vi "36DUT Plot Subvi Ver1.0.vi"(6 "Plot":T1(ring), 7 "No of Rows":i32=10496, 8 "error in (no error)":errorcluster, 9 "No of DUT":i32=16, 10 "Bank":enum16{"C1", "C2", "C3"}(ring), 11 "file path (dialog if empty)":path) -> (0 "error out":errorcluster, 3 "Delta C_Min Plot":dbl[][](graph) caption="(Y) Multi Plot 2")   [LabVIEW 2012]
uses:
  <vilib>/Utility/file.llb/Read From Spreadsheet File (string).vi
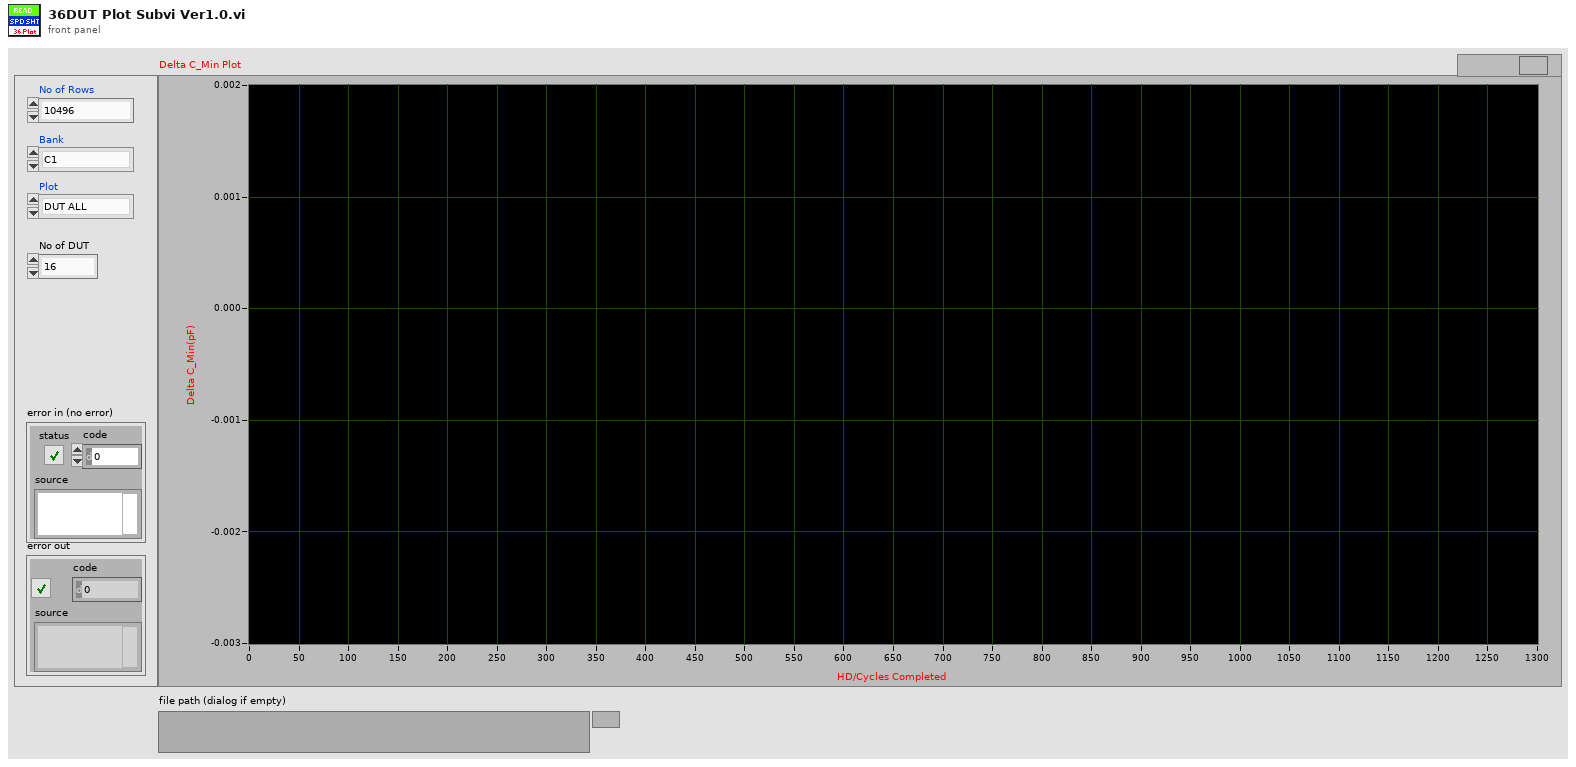
[diagram p1: front panel]
types:
  T1 = enum16{"DUT ALL", "DUT 01", "DUT 02", "DUT 03", "DUT 04", "DUT 05", "DUT 06", "DUT 07", "DUT 08", "DUT 09", "DUT 10", "DUT 11", "DUT 12", "DUT 13", "DUT 14", "DUT 15", "DUT 16", "DUT 17", "DUT 18", "DUT 19", "DUT 20", "DUT 21", "DUT 22", "DUT 23", "DUT 24", "DUT 25", "DUT 26", "DUT 27", "DUT 28", "DUT 29", "DUT 30", "DUT 31", "DUT 32", "DUT 33", "DUT 34", "DUT 35", "DUT 36"}
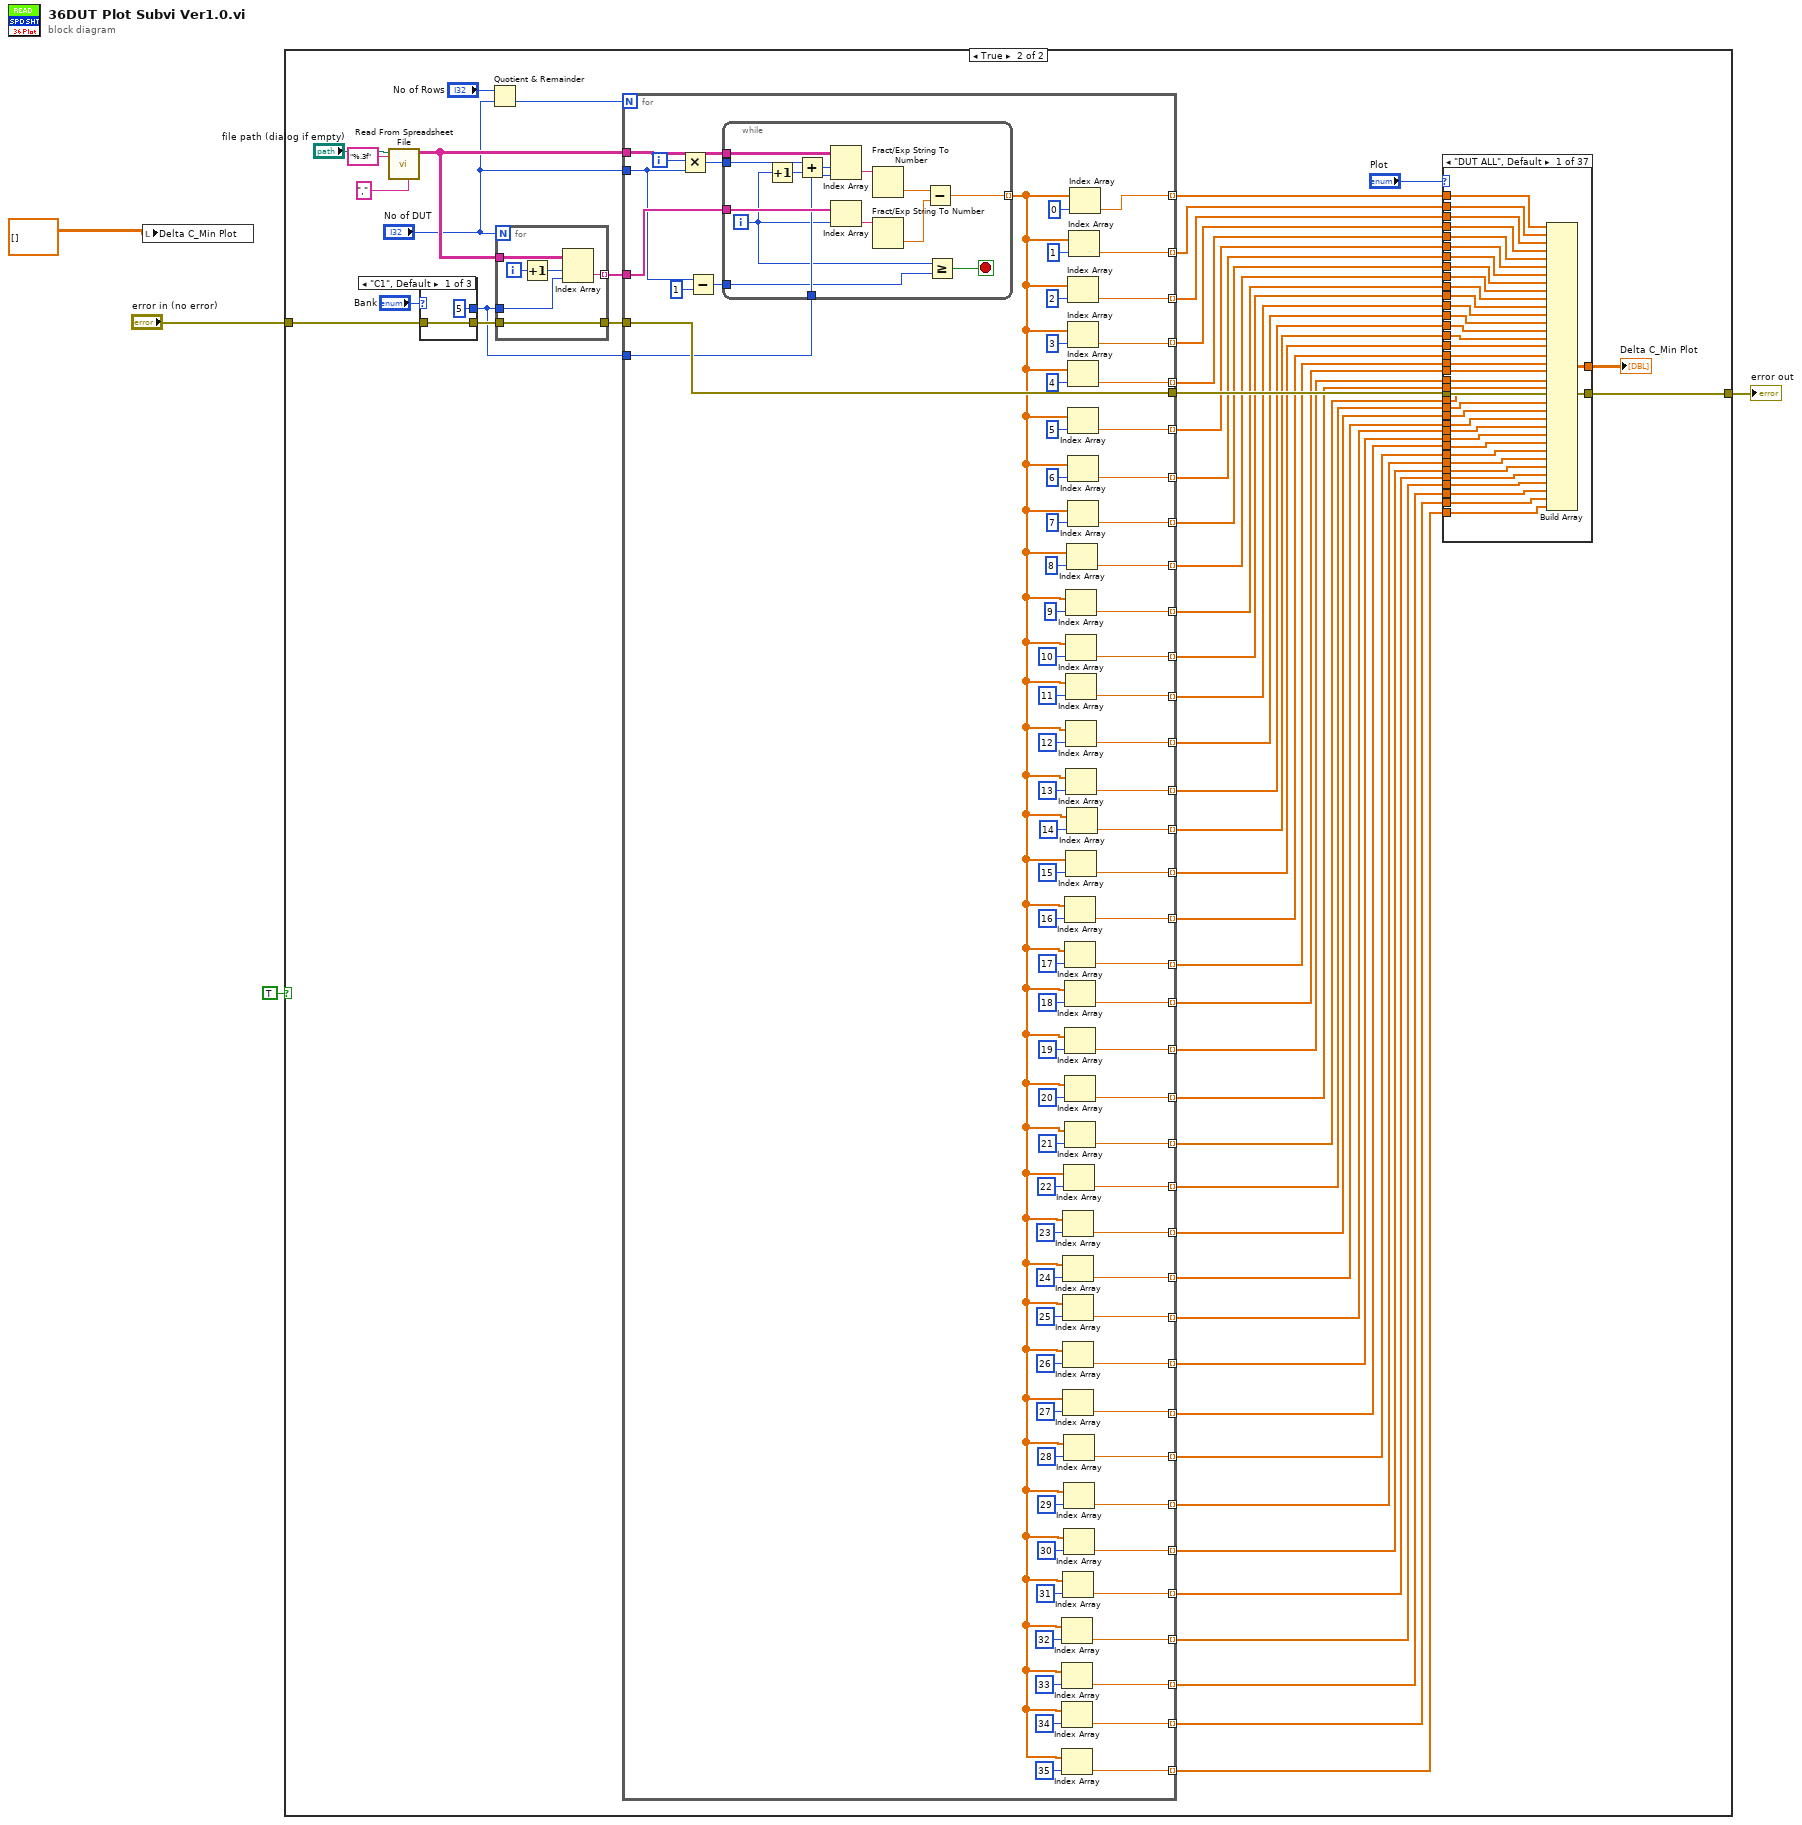
[diagram p0: block diagram]
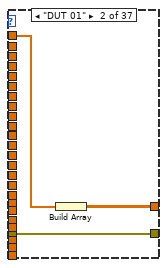
[diagram p3: hidden frame]
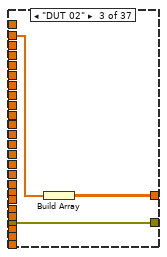
[diagram p4: hidden frame]
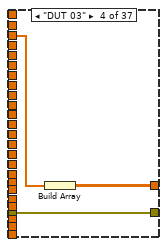
[diagram p5: hidden frame]
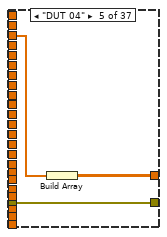
[diagram p6: hidden frame]
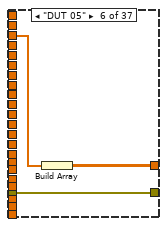
[diagram p7: hidden frame]
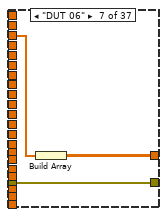
[diagram p8: hidden frame]
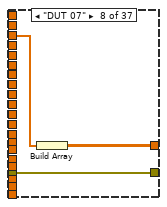
[diagram p9: hidden frame]
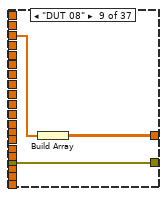
[diagram p10: hidden frame]
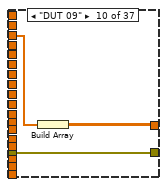
[diagram p11: hidden frame]
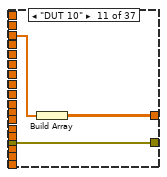
[diagram p12: hidden frame]
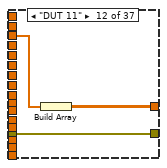
[diagram p13: hidden frame]
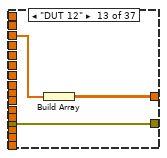
[diagram p14: hidden frame]
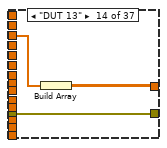
[diagram p15: hidden frame]
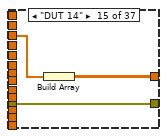
[diagram p16: hidden frame]
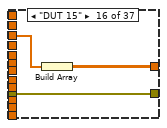
[diagram p17: hidden frame]
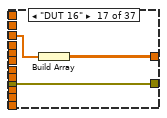
[diagram p18: hidden frame]
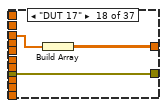
[diagram p19: hidden frame]
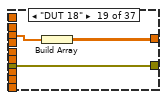
[diagram p20: hidden frame]
diagram:
  n1 = local write "Delta C_Min Plot"(dbl[][] []) -> ()
  n2 = case shown="True" TRUE {
    tunnel: "error in (no error)" -> [w5 w48]
    tunnel: [w5 w42] -> w3
    frame False {
    }
    frame True {
      n3 = call-poly <vilib>:"Read From Spreadsheet File.vi"("delimiter (\\t)"="," ("delimiter (\\t)"), "format (%s)"="%.3f" ("format (%.3f)"), "file path (dialog if empty)"="file path (dialog if empty)") -> ("all rows"=w56:string[][])  [unwired: 4 in, 4 out]
      n4 = case shown="\"C1\", Default" "Bank" {
        tunnel: [5 40 75] -> w44
        tunnel: [w205 w207 w209] -> w45
        tunnel: w48 -> [w205 w207 w209]
        frame "C1", Default {
        }
        frame "C2" {
        }
        frame "C3" {
        }
      }
      n5 = Quotient & Remainder(x="No of Rows", y="No of DUT") -> (floor(x/y)=w52:i32)  [unwired: 1 out]
      n6 = for {
        N: "No of DUT" -> [_]
        tunnel: w56 -> [w312]
        tunnel: [w311] -> w55 mode=indexing
        tunnel: w44 -> [w307]
        tunnel: [w308] -> w47
        tunnel: w45 -> [w308]
        i -> [w310]
        n7 = Increment(x=w310) -> (x+1=w309:i32)
        n8 = Index Array(array=w312, index (row)=w309, index (col)=w307) -> (element=w311:string)
      }
      n9 = for {
        N: w52 -> [_]
        tunnel: w56 -> [w289]
        tunnel: w55 -> [w288]
        tunnel: [w257] -> w50 mode=indexing
        tunnel: w47 -> [w292]
        tunnel: [w292] -> w46
        tunnel: w44 -> [w287]
        tunnel: [w284] -> w41 mode=indexing
        tunnel: [w248] -> w40 mode=indexing
        tunnel: [w247] -> w39 mode=indexing
        tunnel: [w246] -> w37 mode=indexing
        tunnel: [w245] -> w36 mode=indexing
        tunnel: [w244] -> w35 mode=indexing
        tunnel: [w243] -> w34 mode=indexing
        tunnel: [w242] -> w33 mode=indexing
        tunnel: [w241] -> w32 mode=indexing
        tunnel: [w240] -> w31 mode=indexing
        tunnel: [w239] -> w30 mode=indexing
        tunnel: [w238] -> w29 mode=indexing
        tunnel: [w237] -> w28 mode=indexing
        tunnel: [w236] -> w27 mode=indexing
        tunnel: [w235] -> w26 mode=indexing
        tunnel: [w234] -> w25 mode=indexing
        tunnel: [w233] -> w24 mode=indexing
        tunnel: [w232] -> w23 mode=indexing
        tunnel: [w231] -> w22 mode=indexing
        tunnel: [w230] -> w21 mode=indexing
        tunnel: [w229] -> w20 mode=indexing
        tunnel: [w228] -> w19 mode=indexing
        tunnel: [w227] -> w18 mode=indexing
        tunnel: [w226] -> w17 mode=indexing
        tunnel: [w225] -> w16 mode=indexing
        tunnel: [w224] -> w15 mode=indexing
        tunnel: [w223] -> w14 mode=indexing
        tunnel: [w222] -> w13 mode=indexing
        tunnel: [w221] -> w12 mode=indexing
        tunnel: [w220] -> w11 mode=indexing
        tunnel: [w219] -> w10 mode=indexing
        tunnel: [w218] -> w9 mode=indexing
        tunnel: [w217] -> w8 mode=indexing
        tunnel: [w216] -> w7 mode=indexing
        tunnel: [w214] -> w38 mode=indexing
        tunnel: "No of DUT" -> [w212]
        i -> [w291]
        n10 = Multiply(x=w291, y=w212) -> (x*y=w290:i32)
        n11 = Subtract(x=w212, y=1) -> (x-y=w211:i32)
        n12 = while {
          tunnel: w290 -> [w301]
          tunnel: w289 -> [w300]
          tunnel: w288 -> [w299]
          tunnel: w287 -> [w298]
          tunnel: [w294] -> w215 mode=indexing
          tunnel: w211 -> [w293]
          i -> [w295]
          stop <- w296 stop-if-true
          n13 = Increment(x=w295) -> (x+1=w297:i32)
          n14 = Add(x=w301, y=w297) -> (x+y=w302:i32)
          n15 = Index Array(array=w300, index (row)=w302, index (col)=w298) -> (element=w306:string)
          n16 = Index Array(array=w299, index=w295) -> (element=w305:string)
          n17 = Fract/Exp String To Number(string=w306) -> (number=w304:dbl)  [unwired: 3 in, 1 out]
          n18 = Fract/Exp String To Number(string=w305) -> (number=w303:dbl)  [unwired: 3 in, 1 out]
          n19 = Subtract(x=w304, y=w303) -> (x-y=w294:dbl)
          n20 = Greater Or Equal?(x=w295, y=w293) -> (x >= y?=w296:bool)
        }
        n21 = Index Array(array=w215, index=32) -> (element=w219:dbl)
        n22 = Index Array(array=w215, index=33) -> (element=w218:dbl)
        n23 = Index Array(array=w215, index=34) -> (element=w217:dbl)
        n24 = Index Array(array=w215, index=35) -> (element=w216:dbl)
        n25 = Index Array(array=w215, index=23) -> (element=w228:dbl)
        n26 = Index Array(array=w215, index=24) -> (element=w227:dbl)
        n27 = Index Array(array=w215, index=25) -> (element=w226:dbl)
        n28 = Index Array(array=w215, index=26) -> (element=w225:dbl)
        n29 = Index Array(array=w215, index=27) -> (element=w224:dbl)
        n30 = Index Array(array=w215, index=31) -> (element=w220:dbl)
        n31 = Index Array(array=w215, index=22) -> (element=w229:dbl)
        n32 = Index Array(array=w215, index=28) -> (element=w223:dbl)
        n33 = Index Array(array=w215, index=29) -> (element=w222:dbl)
        n34 = Index Array(array=w215, index=30) -> (element=w221:dbl)
        n35 = Index Array(array=w215, index=16) -> (element=w235:dbl)
        n36 = Index Array(array=w215, index=17) -> (element=w234:dbl)
        n37 = Index Array(array=w215, index=18) -> (element=w233:dbl)
        n38 = Index Array(array=w215, index=19) -> (element=w232:dbl)
        n39 = Index Array(array=w215, index=20) -> (element=w231:dbl)
        n40 = Index Array(array=w215, index=21) -> (element=w230:dbl)
        n41 = Index Array(array=w215, index=9) -> (element=w242:dbl)
        n42 = Index Array(array=w215, index=10) -> (element=w241:dbl)
        n43 = Index Array(array=w215, index=11) -> (element=w240:dbl)
        n44 = Index Array(array=w215, index=12) -> (element=w239:dbl)
        n45 = Index Array(array=w215, index=13) -> (element=w238:dbl)
        n46 = Index Array(array=w215, index=15) -> (element=w236:dbl)
        n47 = Index Array(array=w215, index=8) -> (element=w243:dbl)
        n48 = Index Array(array=w215, index=14) -> (element=w237:dbl)
        n49 = Index Array(array=w215, index=2) -> (element=w248:dbl)
        n50 = Index Array(array=w215, index=3) -> (element=w247:dbl)
        n51 = Index Array(array=w215, index=4) -> (element=w214:dbl)
        n52 = Index Array(array=w215, index=5) -> (element=w246:dbl)
        n53 = Index Array(array=w215, index=6) -> (element=w245:dbl)
        n54 = Index Array(array=w215, index=7) -> (element=w244:dbl)
        n55 = Index Array(array=w215, index=1) -> (element=w284:dbl)
        n56 = Index Array(array=w215, index=0) -> (element=w257:dbl)
      }
      n57 = case shown="\"DUT ALL\", Default" "Plot" {
        tunnel: w50 -> [w60 w99 _ _ _ _ _ _ _ _ _ _ _ _ _ _ _ _ _ _ _ _ _ _ _ _ _ _ _ _ _ _ _ _ _ _ _]
        tunnel: w41 -> [w94 _ w101 _ _ _ _ _ _ _ _ _ _ _ _ _ _ _ _ _ _ _ _ _ _ _ _ _ _ _ _ _ _ _ _ _ _]
        tunnel: w40 -> [w93 _ _ w105 _ _ _ _ _ _ _ _ _ _ _ _ _ _ _ _ _ _ _ _ _ _ _ _ _ _ _ _ _ _ _ _ _]
        tunnel: w39 -> [w92 _ _ _ w107 _ _ _ _ _ _ _ _ _ _ _ _ _ _ _ _ _ _ _ _ _ _ _ _ _ _ _ _ _ _ _ _]
        tunnel: w38 -> [w91 _ _ _ _ w111 _ _ _ _ _ _ _ _ _ _ _ _ _ _ _ _ _ _ _ _ _ _ _ _ _ _ _ _ _ _ _]
        tunnel: w37 -> [w90 _ _ _ _ _ w113 _ _ _ _ _ _ _ _ _ _ _ _ _ _ _ _ _ _ _ _ _ _ _ _ _ _ _ _ _ _]
        tunnel: w36 -> [w89 _ _ _ _ _ _ w116 _ _ _ _ _ _ _ _ _ _ _ _ _ _ _ _ _ _ _ _ _ _ _ _ _ _ _ _ _]
        tunnel: w35 -> [w88 _ _ _ _ _ _ _ w120 _ _ _ _ _ _ _ _ _ _ _ _ _ _ _ _ _ _ _ _ _ _ _ _ _ _ _ _]
        tunnel: w34 -> [w87 _ _ _ _ _ _ _ _ w123 _ _ _ _ _ _ _ _ _ _ _ _ _ _ _ _ _ _ _ _ _ _ _ _ _ _ _]
        tunnel: w33 -> [w86 _ _ _ _ _ _ _ _ _ w126 _ _ _ _ _ _ _ _ _ _ _ _ _ _ _ _ _ _ _ _ _ _ _ _ _ _]
        tunnel: w32 -> [w85 _ _ _ _ _ _ _ _ _ _ w129 _ _ _ _ _ _ _ _ _ _ _ _ _ _ _ _ _ _ _ _ _ _ _ _ _]
        tunnel: w31 -> [w84 _ _ _ _ _ _ _ _ _ _ _ w132 _ _ _ _ _ _ _ _ _ _ _ _ _ _ _ _ _ _ _ _ _ _ _ _]
        tunnel: w30 -> [w83 _ _ _ _ _ _ _ _ _ _ _ _ w135 _ _ _ _ _ _ _ _ _ _ _ _ _ _ _ _ _ _ _ _ _ _ _]
        tunnel: w29 -> [w82 _ _ _ _ _ _ _ _ _ _ _ _ _ w138 _ _ _ _ _ _ _ _ _ _ _ _ _ _ _ _ _ _ _ _ _ _]
        tunnel: w28 -> [w81 _ _ _ _ _ _ _ _ _ _ _ _ _ _ w141 _ _ _ _ _ _ _ _ _ _ _ _ _ _ _ _ _ _ _ _ _]
        tunnel: w27 -> [w80 _ _ _ _ _ _ _ _ _ _ _ _ _ _ _ w143 _ _ _ _ _ _ _ _ _ _ _ _ _ _ _ _ _ _ _ _]
        tunnel: [w96 w98 w102 w104 w108 w110 w114 w117 w119 w122 w125 w128 w131 w134 w137 w140 w144 w145 w149 w152 w155 w158 w161 w164 w167 w170 w173 w176 w179 w182 w185 w188 w191 w194 w197 w200 w203] -> w49
        tunnel: w46 -> [w95 w97 w100 w103 w106 w109 w112 w115 w118 w121 w124 w127 w130 w133 w136 w139 w142 w147 w150 w153 w156 w159 w162 w165 w168 w171 w174 w177 w180 w183 w186 w189 w192 w195 w198 w201 w204]
        tunnel: [w95 w97 w100 w103 w106 w109 w112 w115 w118 w121 w124 w127 w130 w133 w136 w139 w142 w147 w150 w153 w156 w159 w162 w165 w168 w171 w174 w177 w180 w183 w186 w189 w192 w195 w198 w201 w204] -> w42
        tunnel: w26 -> [w79 _ _ _ _ _ _ _ _ _ _ _ _ _ _ _ _ w146 _ _ _ _ _ _ _ _ _ _ _ _ _ _ _ _ _ _ _]
        tunnel: w25 -> [w78 _ _ _ _ _ _ _ _ _ _ _ _ _ _ _ _ _ w148 _ _ _ _ _ _ _ _ _ _ _ _ _ _ _ _ _ _]
        tunnel: w24 -> [w77 _ _ _ _ _ _ _ _ _ _ _ _ _ _ _ _ _ _ w151 _ _ _ _ _ _ _ _ _ _ _ _ _ _ _ _ _]
        tunnel: w23 -> [w76 _ _ _ _ _ _ _ _ _ _ _ _ _ _ _ _ _ _ _ w154 _ _ _ _ _ _ _ _ _ _ _ _ _ _ _ _]
        tunnel: w22 -> [w75 _ _ _ _ _ _ _ _ _ _ _ _ _ _ _ _ _ _ _ _ w157 _ _ _ _ _ _ _ _ _ _ _ _ _ _ _]
        tunnel: w21 -> [w74 _ _ _ _ _ _ _ _ _ _ _ _ _ _ _ _ _ _ _ _ _ w160 _ _ _ _ _ _ _ _ _ _ _ _ _ _]
        tunnel: w20 -> [w73 _ _ _ _ _ _ _ _ _ _ _ _ _ _ _ _ _ _ _ _ _ _ w163 _ _ _ _ _ _ _ _ _ _ _ _ _]
        tunnel: w19 -> [w72 _ _ _ _ _ _ _ _ _ _ _ _ _ _ _ _ _ _ _ _ _ _ _ w166 _ _ _ _ _ _ _ _ _ _ _ _]
        tunnel: w18 -> [w71 _ _ _ _ _ _ _ _ _ _ _ _ _ _ _ _ _ _ _ _ _ _ _ _ w169 _ _ _ _ _ _ _ _ _ _ _]
        tunnel: w17 -> [w70 _ _ _ _ _ _ _ _ _ _ _ _ _ _ _ _ _ _ _ _ _ _ _ _ _ w172 _ _ _ _ _ _ _ _ _ _]
        tunnel: w16 -> [w69 _ _ _ _ _ _ _ _ _ _ _ _ _ _ _ _ _ _ _ _ _ _ _ _ _ _ w175 _ _ _ _ _ _ _ _ _]
        tunnel: w15 -> [w68 _ _ _ _ _ _ _ _ _ _ _ _ _ _ _ _ _ _ _ _ _ _ _ _ _ _ _ w178 _ _ _ _ _ _ _ _]
        tunnel: w14 -> [w67 _ _ _ _ _ _ _ _ _ _ _ _ _ _ _ _ _ _ _ _ _ _ _ _ _ _ _ _ w181 _ _ _ _ _ _ _]
        tunnel: w13 -> [w66 _ _ _ _ _ _ _ _ _ _ _ _ _ _ _ _ _ _ _ _ _ _ _ _ _ _ _ _ _ w184 _ _ _ _ _ _]
        tunnel: w12 -> [w65 _ _ _ _ _ _ _ _ _ _ _ _ _ _ _ _ _ _ _ _ _ _ _ _ _ _ _ _ _ _ w187 _ _ _ _ _]
        tunnel: w11 -> [w64 _ _ _ _ _ _ _ _ _ _ _ _ _ _ _ _ _ _ _ _ _ _ _ _ _ _ _ _ _ _ _ w190 _ _ _ _]
        tunnel: w10 -> [w63 _ _ _ _ _ _ _ _ _ _ _ _ _ _ _ _ _ _ _ _ _ _ _ _ _ _ _ _ _ _ _ _ w193 _ _ _]
        tunnel: w9 -> [w62 _ _ _ _ _ _ _ _ _ _ _ _ _ _ _ _ _ _ _ _ _ _ _ _ _ _ _ _ _ _ _ _ _ w196 _ _]
        tunnel: w8 -> [w61 _ _ _ _ _ _ _ _ _ _ _ _ _ _ _ _ _ _ _ _ _ _ _ _ _ _ _ _ _ _ _ _ _ _ w199 _]
        tunnel: w7 -> [w59 _ _ _ _ _ _ _ _ _ _ _ _ _ _ _ _ _ _ _ _ _ _ _ _ _ _ _ _ _ _ _ _ _ _ _ w202]
        frame "DUT ALL", Default {
          n58 = Build Array(w60, w94, w93, w92, w91, w90, w89, w88, w87, w86, w85, w84, w83, w82, w81, w80, w79, w78, w77, w76, w75, w74, w73, w72, w71, w70, w69, w68, w67, w66, w65, w64, w63, w62, w61, w59) -> (w96:dbl[][])
        }
        frame "DUT 01" {
          n59 = Build Array(w99) -> (w98:dbl[][])
        }
        frame "DUT 02" {
          n60 = Build Array(w101) -> (w102:dbl[][])
        }
        frame "DUT 03" {
          n61 = Build Array(w105) -> (w104:dbl[][])
        }
        frame "DUT 04" {
          n62 = Build Array(w107) -> (w108:dbl[][])
        }
        frame "DUT 05" {
          n63 = Build Array(w111) -> (w110:dbl[][])
        }
        frame "DUT 06" {
          n64 = Build Array(w113) -> (w114:dbl[][])
        }
        frame "DUT 07" {
          n65 = Build Array(w116) -> (w117:dbl[][])
        }
        frame "DUT 08" {
          n66 = Build Array(w120) -> (w119:dbl[][])
        }
        frame "DUT 09" {
          n67 = Build Array(w123) -> (w122:dbl[][])
        }
        frame "DUT 10" {
          n68 = Build Array(w126) -> (w125:dbl[][])
        }
        frame "DUT 11" {
          n69 = Build Array(w129) -> (w128:dbl[][])
        }
        frame "DUT 12" {
          n70 = Build Array(w132) -> (w131:dbl[][])
        }
        frame "DUT 13" {
          n71 = Build Array(w135) -> (w134:dbl[][])
        }
        frame "DUT 14" {
          n72 = Build Array(w138) -> (w137:dbl[][])
        }
        frame "DUT 15" {
          n73 = Build Array(w141) -> (w140:dbl[][])
        }
        frame "DUT 16" {
          n74 = Build Array(w143) -> (w144:dbl[][])
        }
        frame "DUT 17" {
          n75 = Build Array(w146) -> (w145:dbl[][])
        }
        frame "DUT 18" {
          n76 = Build Array(w148) -> (w149:dbl[][])
        }
        frame "DUT 19" {
          n77 = Build Array(w151) -> (w152:dbl[][])
        }
        frame "DUT 20" {
          n78 = Build Array(w154) -> (w155:dbl[][])
        }
        frame "DUT 21" {
          n79 = Build Array(w157) -> (w158:dbl[][])
        }
        frame "DUT 22" {
          n80 = Build Array(w160) -> (w161:dbl[][])
        }
        frame "DUT 23" {
          n81 = Build Array(w163) -> (w164:dbl[][])
        }
        frame "DUT 24" {
          n82 = Build Array(w166) -> (w167:dbl[][])
        }
        frame "DUT 25" {
          n83 = Build Array(w169) -> (w170:dbl[][])
        }
        frame "DUT 26" {
          n84 = Build Array(w172) -> (w173:dbl[][])
        }
        frame "DUT 27" {
          n85 = Build Array(w175) -> (w176:dbl[][])
        }
        frame "DUT 28" {
          n86 = Build Array(w178) -> (w179:dbl[][])
        }
        frame "DUT 29" {
          n87 = Build Array(w181) -> (w182:dbl[][])
        }
        frame "DUT 30" {
          n88 = Build Array(w184) -> (w185:dbl[][])
        }
        frame "DUT 31" {
          n89 = Build Array(w187) -> (w188:dbl[][])
        }
        frame "DUT 32" {
          n90 = Build Array(w190) -> (w191:dbl[][])
        }
        frame "DUT 33" {
          n91 = Build Array(w193) -> (w194:dbl[][])
        }
        frame "DUT 34" {
          n92 = Build Array(w196) -> (w197:dbl[][])
        }
        frame "DUT 35" {
          n93 = Build Array(w199) -> (w200:dbl[][])
        }
        frame "DUT 36" {
          n94 = Build Array(w202) -> (w203:dbl[][])
        }
      }
      "Delta C_Min Plot" <- w49
    }
  }
  "error out" <- w3
